vi "Evaluate.vi"(8 "error in (no error)":errorcluster, 10 "Trigger Data":dbl[](array[numeric]), 11 "Trigger in":refnum<class "Trigger.lvclass">) -> (0 "error out":errorcluster, 2 "Trigger":bool, 3 "Trigger out":refnum<class "Trigger.lvclass">)   [LabVIEW 2015, in "Trigger.lvclass"]
doc: "Evaluates the trigger data and returns whether the specified trigger condition was met."
uses:
  Trigger.lvclass
  Trigger.lvclass/Trigger.ctl
  Digital Edge Trigger/Digital Edge Trigger.lvclass
  Digital Edge Trigger/Digital Edge Trigger.lvclass/Digital Edge Trigger.ctl
  Analog Edge Trigger/Analog Edge Trigger.lvclass
  Analog Edge Trigger/Analog Edge Trigger.lvclass/Analog Edge Trigger.ctl
  Value Change Trigger/Value Change Trigger.lvclass
  Value Change Trigger/Value Change Trigger.lvclass/Value Change Trigger.ctl
  Boolean Evaluation Trigger/Boolean Evaluation Trigger.lvclass
  Boolean Evaluation Trigger/Boolean Evaluation Trigger.lvclass/Boolean Evaluation Trigger.ctl
  In Range Trigger/In Range Trigger.lvclass
  Default Trigger/Default Trigger.lvclass
  Default Trigger/Default Trigger.lvclass/Default Trigger.ctl
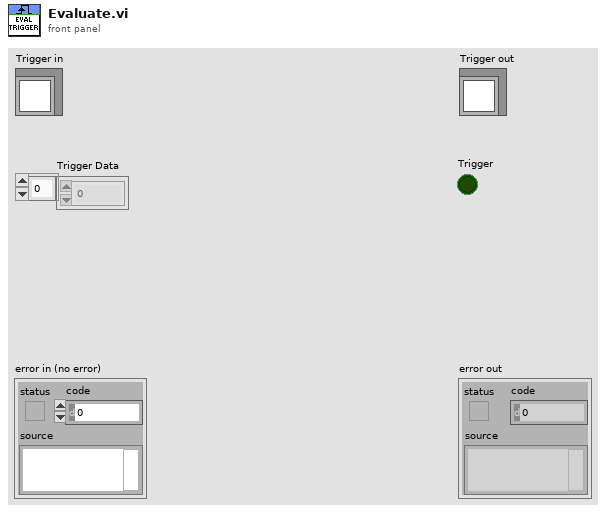
[diagram p1: front panel]
types:
  T1 = typedef "Trigger.lvclass/Trigger Type.ctl" = enum16{"Default", "Digital Edge", "Analog Edge", "In Range", "Value Change", "Boolean Evaluation"}
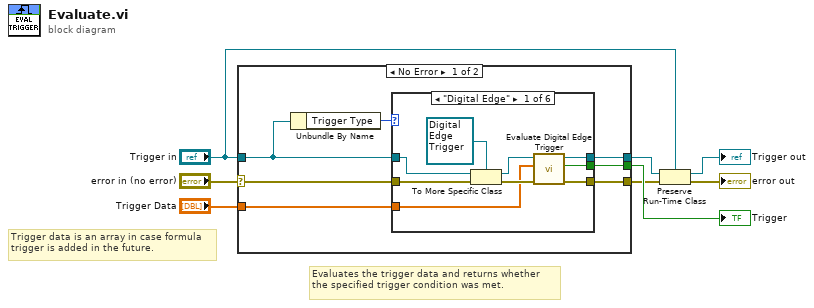
[diagram p0: block diagram]
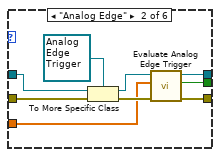
[diagram p2: hidden frame]
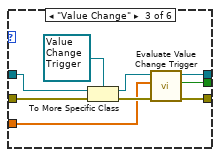
[diagram p3: hidden frame]
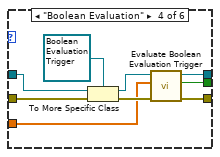
[diagram p4: hidden frame]
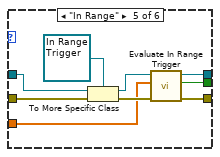
[diagram p5: hidden frame]
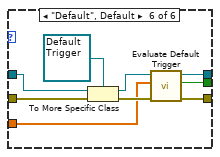
[diagram p6: hidden frame]
diagram:
  # "Trigger data is an array in case formula\ntrigger is added in the future."
  # "Evaluates the trigger data and returns whether the specified trigger condition was met."
  n1 = case shown="No Error" "error in (no error)" {
    selector: "error in (no error)" -> [w12 w70]
    tunnel: "Trigger in" -> [w14 w71]
    tunnel: [w13 w71] -> w3
    tunnel: [w11 w70] -> w5
    tunnel: "Trigger Data" -> [w10 _]
    tunnel: [w9 _] -> w6
    frame No Error {
      n2 = Unbundle By Name(w14) -> ("Trigger Type"=w15:T1)
      n3 = case shown="\"Digital Edge\"" w15 {
        tunnel: w14 -> [w22 w33 w42 w51 w60 w69]
        tunnel: [w24 w27 w36 w45 w54 w63] -> w13
        tunnel: [w19 w29 w38 w47 w56 w65] -> w11
        tunnel: w12 -> [w18 w32 w41 w50 w59 w68]
        tunnel: w10 -> [w17 w26 w35 w44 w53 w62]
        tunnel: [w16 w25 w34 w43 w52 w61] -> w9
        frame "Digital Edge" {
          n4 = To More Specific Class(target class=refnum<class "Digital Edge Trigger.lvclass"> refnum ("Digital Edge Trigger.lvclass"), reference=w22, error in=w18) -> (specific class reference=w20:refnum<class "Digital Edge Trigger.lvclass">, error out=w23:errorcluster)
          n5 = call "Evaluate Digital Edge Trigger.vi"("error in (no error)"=w23, "Trigger Data"=w17, "Digital Edge Trigger in"=w20) -> ("error out"=w19:errorcluster, "Trigger"=w16:bool, "Digital Edge Trigger out"=w24:refnum<class "Digital Edge Trigger.lvclass">)  [unwired: 6 in]
        }
        frame "Analog Edge" {
          n6 = To More Specific Class(target class=refnum<class "Analog Edge Trigger.lvclass"> refnum ("Analog Edge Trigger.lvclass"), reference=w33, error in=w32) -> (specific class reference=w28:refnum<class "Analog Edge Trigger.lvclass">, error out=w30:errorcluster)
          n7 = call "Evaluate Analog Edge Trigger.vi"("error in (no error)"=w30, "Trigger Data"=w26, "Analog Edge Trigger in"=w28) -> ("error out"=w29:errorcluster, "Trigger"=w25:bool, "Analog Edge Trigger out"=w27:refnum<class "Analog Edge Trigger.lvclass">)  [unwired: 6 in]
        }
        frame "Value Change" {
          n8 = To More Specific Class(target class=refnum<class "Value Change Trigger.lvclass"> refnum ("Value Change Trigger.lvclass"), reference=w42, error in=w41) -> (specific class reference=w37:refnum<class "Value Change Trigger.lvclass">, error out=w39:errorcluster)
          n9 = call "Evaluate Value Change Trigger.vi"("error in (no error)"=w39, "Trigger Data"=w35, "Value Change Trigger in"=w37) -> ("error out"=w38:errorcluster, "Trigger"=w34:bool, "Value Change Trigger out"=w36:refnum<class "Value Change Trigger.lvclass">)  [unwired: 6 in]
        }
        frame "Boolean Evaluation" {
          n10 = To More Specific Class(target class=refnum<class "Boolean Evaluation Trigger.lvclass"> refnum ("Boolean Evaluation Trigger.lvclass"), reference=w51, error in=w50) -> (specific class reference=w46:refnum<class "Boolean Evaluation Trigger.lvclass">, error out=w48:errorcluster)
          n11 = call "Evaluate Boolean Evaluation Trigger.vi"("error in (no error)"=w48, "Trigger Data"=w44, "Boolean Evaluation Trigger in"=w46) -> ("error out"=w47:errorcluster, "Trigger"=w43:bool, "Boolean Evaluation Trigger out"=w45:refnum<class "Boolean Evaluation Trigger.lvclass">)  [unwired: 6 in]
        }
        frame "In Range" {
          n12 = To More Specific Class(target class=refnum<class "In Range Trigger.lvclass"> refnum ("In Range Trigger.lvclass"), reference=w60, error in=w59) -> (specific class reference=w55:refnum<class "In Range Trigger.lvclass">, error out=w57:errorcluster)
          n13 = call "Evaluate In Range Trigger.vi"("error in (no error)"=w57, "Trigger Data"=w53, "In Range Trigger in"=w55) -> ("error out"=w56:errorcluster, "Trigger"=w52:bool, "In Range Trigger out"=w54:refnum<class "In Range Trigger.lvclass">)  [unwired: 6 in]
        }
        frame "Default", Default {
          n14 = To More Specific Class(target class=refnum<class "Default Trigger.lvclass"> refnum ("Default Trigger.lvclass"), reference=w69, error in=w68) -> (specific class reference=w64:refnum<class "Default Trigger.lvclass">, error out=w66:errorcluster)
          n15 = call "Evaluate Default Trigger.vi"("error in (no error)"=w66, "Trigger Data"=w62, "Default Trigger in"=w64) -> ("error out"=w65:errorcluster, "Trigger"=w61:bool, "Default Trigger out"=w63:refnum<class "Default Trigger.lvclass">)  [unwired: 6 in]
        }
      }
    }
    frame Error {
    }
  }
  "Trigger" <- w6
  n16 = Preserve Run-Time Class(object in=w3, error in=w5, 2:"Trigger in") -> (object out=→"Trigger out":refnum<class "Trigger.lvclass">, error out=→"error out":errorcluster)
